vi "timerfd_create.vi"(8 "error in (no error)":errorcluster, 11 "clock id (monotonic)":enum16{"Realtime", "Monotonic"}(ring)=enum."Monotonic") -> (0 "error out":errorcluster, 3 "timer fd":i32)   [LabVIEW 2016, in "Linux RT IPC.C.lvlib"]
uses:
  Linux RT IPC.C.lvlib
  Controls/functions.ctl
  <vilib>/NI/NI Linux RT Errno/Linux Errno.lvlib
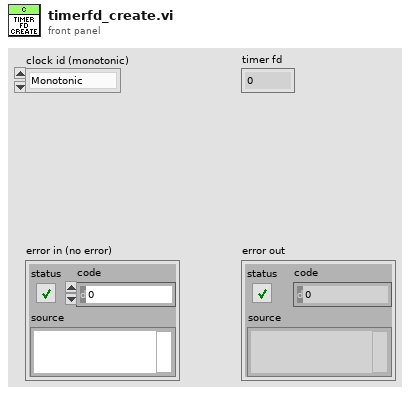
[diagram p1: front panel]
types:
  T1 = typedef "Linux RT IPC.C.lvlib/functions.ctl" = enum16{"unspecified", "close", "epoll_create", "epoll_ctl", "epoll_wait", "fstat", "ftruncate", "mkfifo", "mmap", "munmap", "open", "read", "shm_open", "shm_unlink", "timerfd_create", "timerfd_settime", "timerfd_gettime", "write", "unlink"}
  T2 = typedef "Linux Errno.lvlib/errno.ctl" = enum16{"NO ERROR", "EPERM", "ENOENT", "ESRCH", "EINTR", "EIO", "ENXIO", "E2BIG", "ENOEXEC", "EBADF", "ECHILD", "EAGAIN", "ENOMEM", "EACCES", "EFAULT", "ENOTBLK", "EBUSY", "EEXIST", "EXDEV", "ENODEV", "ENOTDIR", "EISDIR", "EINVAL", "ENFILE", "EMFILE", "ENOTTY", "ETXTBSY", "EFBIG", "ENOSPC", "ESPIPE", "EROFS", "EMLINK", "EPIPE", "EDOM", "ERANGE", "EDADLK", "ENAMETOOLONG", "ENOLCK", "ENOSYS", "ENOTEMPTY", "ELOOP", "EWOULDBLOCK", "ENOMSG", "EIDRM", "ECHRNG", "EL2NSYNC", "EL3HLT", "EL3RST", "ELNRNG", "EUNATCH", "ENOCSI", "EL2HLT", "EBADE", "EBADR", "EXFULL", "ENOANO", "EBADRQC", "EBADSLT", "EDEADLOCK", "EBFONT", "ENOSTR", "ENODATA", "ETIME", "ENOSR", "ENONET", "ENOPKG", "EREMOTE", "ENOLINK", "EADV", "ESRMNT", "ECOMM", "EPROTO", "EMULTIHOP", "EDOTDOT", "EBADMSG", "EOVERFLOW", "ENOTUNIQ", "EBADFD", "EREMCHG", "ELIBACC", "ELIBBAD", "ELIBSCN", "ELIBMAX", "ELIBEXEC", "ELISEQ", "ERESTART", "ESTRPIPE", "EUSERS", "ENOTSOCK", "EDESTADDRREQ", "EMSGSIZE", "EPROTOTYPE", "ENOPROTOOPT", "EPROTONOSUPPORT", "ESOCKTNOSUPPORT", "EOPNOTSUPP", "EPFNOSUPPORT", "EAFNOSUPPORT", "EADDRINUSE", "EADDRNOTAVAIL", "ENETDOWN", "ENETUNREACH", "ENETRESET", "ECONNABORTED", "ECONNRESET", "ENOBUFS", "EISCONN", "ENOTCONN", "ESHUTDOWN", "ETOOMANYREFS", "ETIMEDOUT", "ECONNREFUSED", "EHOSTDOWN", "EHOSTUNREACH", "EALREADY", "EINPROGRESS", "ESTALE", "EUCLEAN", "ENOTNAM", "ENAVAIL", "EISNAM", "EREMOTEIO", "EDQUOT", "ENOMEDIUM", "EMEDIUMTYPE", "ECANCELED", "ENOKEY", "EKEYEXPIRED", "EKEYREVOKED", "EKEYREJECTED", "EOWNERDEAD", "ENOTRECOVERABLE", "ERFKILL", "EHWPOISON", "UNDEFINED"}
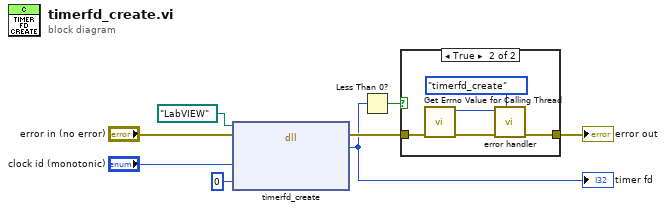
[diagram p0: block diagram]
diagram:
  n1 = dll-call lib="LabVIEW" fn="timerfd_create"(path in=path "LabVIEW", error in="error in (no error)", "clock_id"="clock id (monotonic)", "flags"=u16 0) -> (error out=w7:errorcluster, "return"=w1:i32)  [unwired: 3 in, 1 out]
  "timer fd" <- w1
  n2 = Less Than 0?(x=w1) -> (x < 0?=w5:bool)
  n3 = case shown="True" w5 {
    tunnel: w7 -> [w9 w14]
    tunnel: [w9 w13] -> w6
    frame False {
    }
    frame True {
      n4 = call <vilib>:"Get Errno Value for Calling Thread.vi"("error in (no error)"=w14) -> ("error out"=w11:errorcluster, "errno"=w12:T2)  [unwired: 9 in]
      n5 = call "error handler.vi"("function (unspecified)"=functions."timerfd_create" ("function"), "error in (no error)"=w11, "errno"=w12) -> ("error out"=w13:errorcluster)  [unwired: 8 in]
    }
  }
  "error out" <- w6
